vi "Forward Substatus.vi"(8 "error in (no error)":errorcluster, 10 "Module Substatus":T1, 11 "Module in":refnum<class "Module.lvclass">) -> (0 "error out":errorcluster, 3 "Module out":refnum<class "Module.lvclass">)   [LabVIEW 2020, in "Volatus.lvlib" / "Module.lvclass"]
uses:
  Module.lvclass
  Module Substatus.ctl
  Module.lvclass/Module.ctl
  MessageQ/MessageQ.lvclass/MessageQ.ctl
  MessageQ/MessageQ.lvclass
  Volatus.lvlib
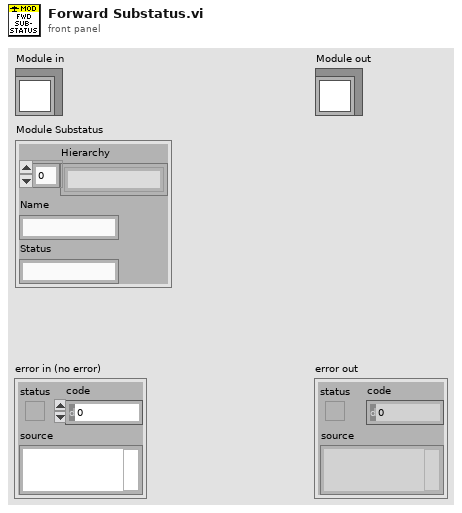
[diagram p1: front panel]
types:
  T1 = typedef "Volatus.lvlib/Module Substatus.ctl" = cluster{"Hierarchy":string[], "Name":string, "Status":string}
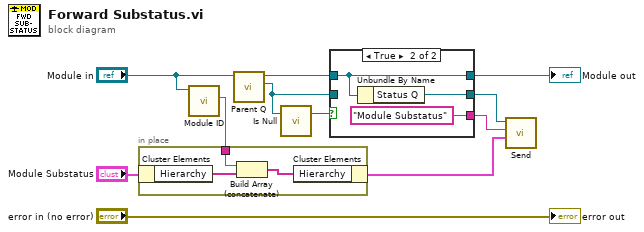
[diagram p0: block diagram]
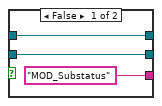
[diagram p2: hidden frame]
diagram:
  n1 = call-dynamic "Module ID.vi"("Module in"="Module in") -> ("Module ID"=w2:string)  [unwired: 10 in]
  n2 = in-place {
    in-place-border: w2 -> [w13]
    n3 = in-place-cluster #1("Module Substatus") -> ("Hierarchy"=w14:string[])
    n4 = Build Array (concatenate)(w13, w14) -> (w12:string[])
    n5 = in-place-cluster #1("Hierarchy"=w12) -> (w1:T1)
  }
  n6 = call "Parent Q.vi"("Module in"="Module in") -> ("Parent Q"=w9:refnum<class "MessageQ.lvclass">, "Module out"=w6:refnum<class "Module.lvclass">)  [unwired: 9 in]
  n7 = call "Is Null.vi"("MessageQ in"=w9) -> ("Null"=w10:bool)  [unwired: 2 in]
  n8 = case shown="True" w10 {
    tunnel: w9 -> [w16 _]
    tunnel: ["MOD_Substatus" ("ID") "Module Substatus" ("ID")] -> w8
    tunnel: [w16 w18] -> w7
    tunnel: w6 -> [w15 w19]
    tunnel: [w15 w19] -> w5
    frame False {
    }
    frame True {
      n9 = Unbundle By Name(w19) -> ("Status Q"=w18:refnum<class "MessageQ.lvclass">)
    }
  }
  "Module out" <- w5
  n10 = call "Send.vi"("Data"=w1, "ID"=w8, "MessageQ in"=w7) -> ()  [unwired: 7 in, 2 out]
  "error out" <- "error in (no error)"
